vi "Append a New Styled Run.vi"(8 "error in (no error)":errorcluster, 9 "Run Type":T1(ring), 10 "Text":string, 11 "xwpfParagraph in":refnum<class "xwpfParagraph.lvclass">) -> (0 "error out":errorcluster, 3 "xwpfParagraph out":refnum<class "xwpfParagraph.lvclass">)   [LabVIEW 2017, in "Word_Specific.lvlib" / "xwpfParagraph.lvclass"]
uses:
  xwpfParagraph.lvclass
  xwpfParagraph.lvclass/xwpfParagraph.ctl
  C:/Users/Neo/Desktop/Dev_Tools_BR/LabVIEW_NPOI/lib/NPOI 2.1.1/NPOI.OOXML.dll
  lib/NPOI 2.1.1/NPOI.OOXML.dll
  xwpfRun/xwpfRun.lvclass
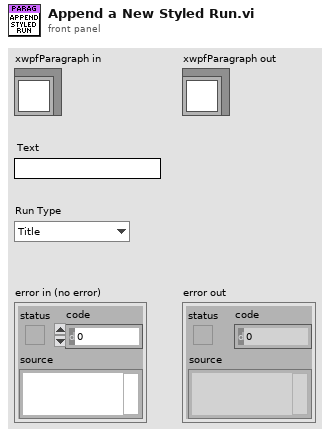
[diagram p1: front panel]
types:
  T1 = enum16{"Title", "Heading 1", "Heading 2", "Heading 3", "Normal", "Figure", "Page Break"}
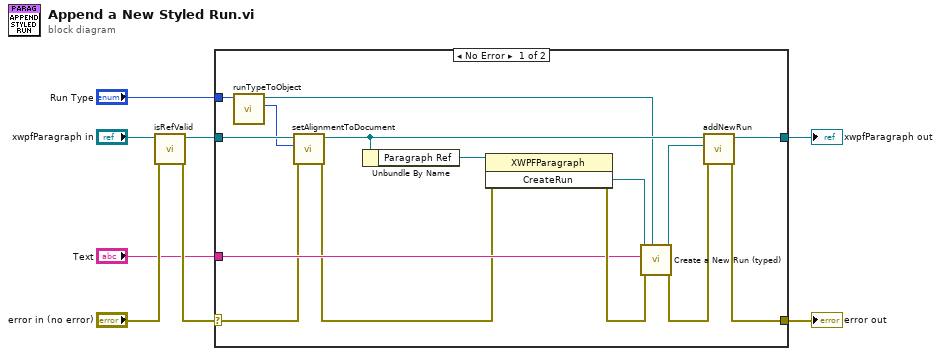
[diagram p0: block diagram]
diagram:
  n1 = call-dynamic "isRefValid.vi"("error in (no error)"="error in (no error)", "xwpfParagraph in"="xwpfParagraph in") -> ("error out"=w3:errorcluster, "xwpfParagraph out"=w5:refnum<class "xwpfParagraph.lvclass">)  [unwired: 8 in]
  n2 = case shown="No Error" w3 {
    selector: w3 -> [w13 w25]
    tunnel: [w15 w25] -> w8
    tunnel: [w18 w24] -> w6
    tunnel: w5 -> [w19 w24]
    tunnel: "Text" -> [w20 _]
    tunnel: "Run Type" -> [w10 _]
    frame No Error {
      n3 = call "runTypeToObject.vi"("Run Type"=w10) -> ("Alignment"=w9:u16, "Run Type Object"=w11:refnum<class "xwpfRun.lvclass">)  [unwired: 9 in]
      n4 = call "setAlignmentToDocument.vi"("error in (no error)"=w13, "Alignment"=w9, "xwpfParagraph in"=w19) -> ("error out"=w12:errorcluster, "xwpfParagraph out"=w14:refnum<class "xwpfParagraph.lvclass">)  [unwired: 7 in]
      n5 = Unbundle By Name(w14) -> ("Paragraph Ref"=w23:refnum<k24>)
      n6 = invoke class="XWPFParagraph" method="CreateRun"(reference=w23, error in=w12) -> (error out=w21:errorcluster, "CreateRun"=w22:refnum<k24>)  [unwired: 1 in, 1 out]
      n7 = call "Create a New Run (typed).vi"("xwpfRun Type"=w11, "error in (no error)"=w21, "Text"=w20, "Run Ref"=w22) -> ("error out"=w16:errorcluster, "xwpfRun out"=w17:refnum<class "xwpfRun.lvclass">)  [unwired: 6 in]
      n8 = call "addNewRun.vi"("error in (no error)"=w16, "New Run"=w17, "xwpfParagraph in"=w14) -> ("error out"=w15:errorcluster, "xwpfParagraph out"=w18:refnum<class "xwpfParagraph.lvclass">)  [unwired: 7 in]
    }
    frame Error {
    }
  }
  "error out" <- w8
  "xwpfParagraph out" <- w6
